vi "CIE-Delete Exemplar Plot.vi"(0 "Mag graph":refnum<vi>, 11 "error in (no error)":errorcluster) -> (15 "error out":errorcluster)   [LabVIEW 2015]
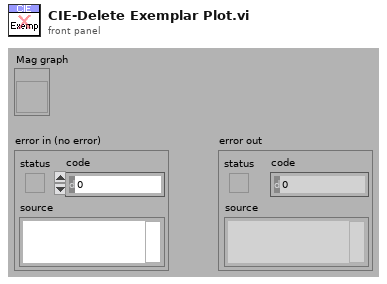
[diagram p1: front panel]
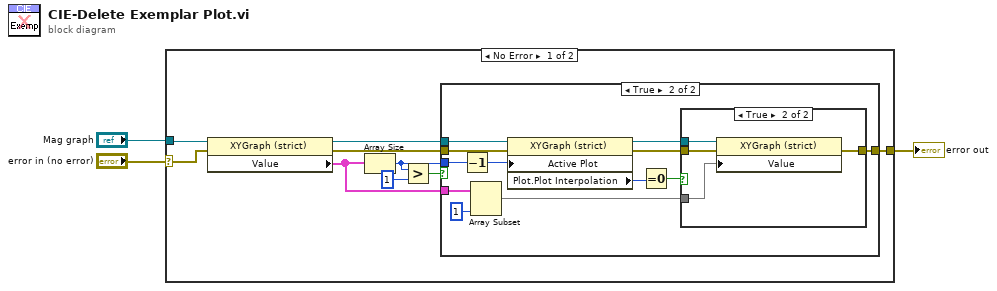
[diagram p0: block diagram]
diagram:
  n1 = case shown="No Error" "error in (no error)" {
    selector: "error in (no error)" -> [w11 w31]
    tunnel: "Mag graph" -> [w12 _]
    tunnel: [w7 w31] -> w1
    frame No Error {
      n2 = property class="XYGraph (strict)"(reference=w12, error in=w11) -> (reference out=w10:refnum<vi>, error out=w9:errorcluster, "Value"=w8:cluster{"PTC Mag":dbl[], "PTC Phase":dbl[]}[])
      n3 = Array Size(array=w8) -> (size(s)=w6:i32)
      n4 = Greater?(x=w6, y=1) -> (0:w5:bool)
      n5 = case shown="True" w5 {
        tunnel: w10 -> [_ w25]
        tunnel: w9 -> [w13 w24]
        tunnel: w6 -> [_ w18]
        tunnel: w8 -> [_ w17]
        tunnel: [w13 w15] -> w7
        frame False {
        }
        frame True {
          n6 = Decrement(x=w18) -> (x-1=w23:i32)
          n7 = Array Subset(array=w17, length=1) -> (w16:cluster{"PTC Mag":dbl[], "PTC Phase":dbl[]}[])  [unwired: 1 in]
          n8 = property class="XYGraph (strict)"(reference=w25, error in=w24, "Active Plot"=w23) -> (reference out=w21:refnum<vi>, error out=w20:errorcluster, "Plot.Plot Interpolation"=w22:u8)
          n9 = Equal To 0?(x=w22) -> (x = 0?=w19:bool)
          n10 = case shown="True" w19 {
            tunnel: w21 -> [_ w30]
            tunnel: w20 -> [w26 w29]
            tunnel: w16 -> [_ w28]
            tunnel: [w26 w27] -> w15
            frame False {
            }
            frame True {
              n11 = property class="XYGraph (strict)"(reference=w30, error in=w29, "Value"=w28) -> (error out=w27:errorcluster)  [unwired: 1 out]
            }
          }
        }
      }
    }
    frame Error {
    }
  }
  "error out" <- w1
